vi "input_pos.vi"(2 "positie":dbl, 3 "VISA in":refnum<visa-resource-name>) -> (0 "error out":errorcluster, 1 "VISA out":refnum<visa-resource-name>)   [LabVIEW 2018]
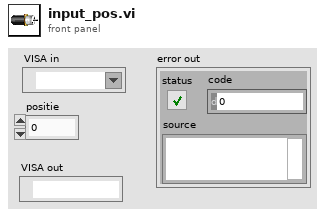
[diagram p1: front panel]
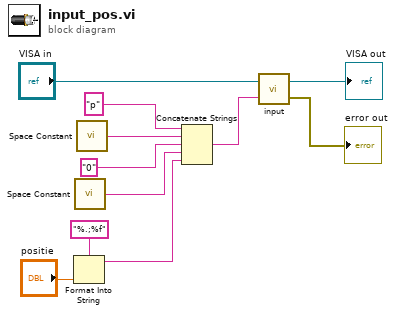
[diagram p0: block diagram]
diagram:
  n1 = Format Into String(format string="%.;%f", "positie") -> (resulting string=w4:string)  [unwired: 2 in, 1 out]
  n2 = call <vilib>:"Space Constant.vi"() -> ("String"=w11:string)
  n3 = call <vilib>:"Space Constant.vi"() -> ("String"=w9:string)
  n4 = Concatenate Strings("p" ("write buffer"), w9, "0", w11, w4) -> (w7:string)
  n5 = call "input.vi"("commando"=w7, "VISA in"="VISA in") -> ("error out"=→"error out":errorcluster, "VISA out"=→"VISA out":refnum<visa-resource-name>)
